vi "Set Rx Monitor Properties.vi"(8 "error in":errorcluster, 10 "session_rx_monitor":T2 {"Strobe" items=["FDX_MON_STROBE_DIS", "FDX_MON_STROBE_STOP", "FDX_MON_STROBE_START"]; "CaptureMode" items=["FDX_MON_SINGLE ", "FDX_MON_CONTINUOUS", "FDX_MON_SELECTIVE", "FDX_MON_RECORDING", "FDX_MON_REROS", "FDX_MON_HMU"]; "DefaultCronoMode" items=["FDX_RX_DEFAULT_ENA_CNT", "FDX_RX_DEFAULT_MON_ENA_ALL", "FDX_RX_DEFAULT_MON_ENA_GOOD"]}, 11 "custom device ref in":T1 format="%.0x") -> (0 "error out":errorcluster, 3 "custom device ref out":T1 format="%.0x")   [LabVIEW 2020, in "AIM ARINC 664 Scripting.lvlib"]
uses:
  AIM ARINC 664 Scripting.lvlib
  <vilib>/NI VeriStand/Custom Device API/Custom Device API.lvlib
  <vilib>/NI VeriStand/Custom Device API/Set Item Property (U32).vi
  Constants.vi
  <vilib>/NI VeriStand/Custom Device API/Custom Device Item Ref.ctl
  Shared/session_rx_monitor.ctl
  Import/AIM ARINC 664 Import.lvlib
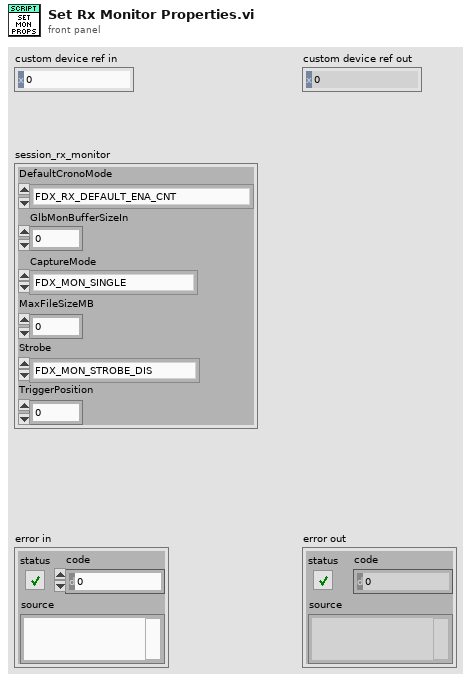
[diagram p1: front panel]
types:
  T1 = typedef "Custom Device API.lvlib/Custom Device Item Ref.ctl" = u64
  T2 = typedef "AIM ARINC 664 Import.lvlib/session_rx_monitor.ctl" = cluster{"DefaultCronoMode":u32, "GlbMonBufferSizeIn":u32, "CaptureMode":u32, "MaxFileSizeMB":u32, "Strobe":u32, "TriggerPosition":u32}
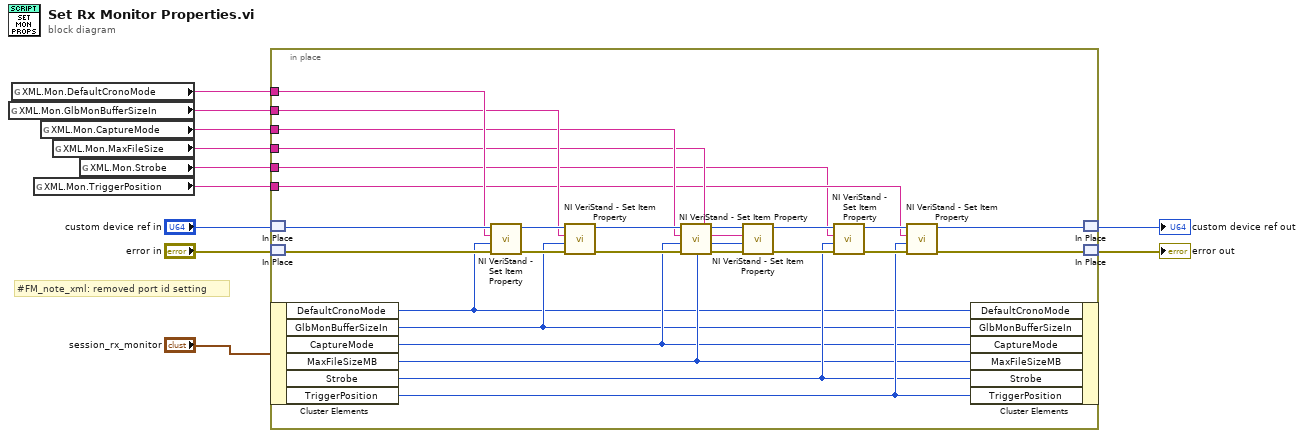
[diagram p0: block diagram]
diagram:
  # "#FM_note_xml: removed port id setting"
  n1 = global read "Constants.vi" "XML.Mon.GlbMonBufferSizeIn"() -> (w5:string)
  n2 = global read "Constants.vi" "XML.Mon.DefaultCronoMode"() -> (w6:string)
  n3 = global read "Constants.vi" "XML.Mon.TriggerPosition"() -> (w2:string)
  n4 = global read "Constants.vi" "XML.Mon.CaptureMode"() -> (w4:string)
  n5 = global read "Constants.vi" "XML.Mon.MaxFileSize"() -> (w3:string)
  n6 = global read "Constants.vi" "XML.Mon.Strobe"() -> (w1:string)
  n7 = in-place {
    in-place-border: w6 -> [w17]
    in-place-border: w5 -> [w16]
    in-place-border: w4 -> [w15]
    in-place-border: w3 -> [w14]
    in-place-border: w2 -> [w13]
    in-place-border: w1 -> [w12]
    n8 = in-place-match #1("custom device ref in") -> (w37:T1)
    n9 = in-place-match #2("error in") -> (w31:errorcluster)
    n10 = in-place-cluster #3("session_rx_monitor") -> ("DefaultCronoMode"=w19:u32, "GlbMonBufferSizeIn"=w20:u32, "CaptureMode"=w21:u32, "MaxFileSizeMB"=w22:u32, "Strobe"=w23:u32, "TriggerPosition"=w24:u32)
    n11 = call-poly <vilib>:"NI VeriStand - Set Item Property.vi"("error in (no error)"=w31, "Value"=w19, "Property Name"=w17, "Item Ref in"=w37) -> ("error out"=w30:errorcluster, "Item Ref out"=w36:T1)  [unwired: 5 in, 1 out]
    n12 = call-poly <vilib>:"NI VeriStand - Set Item Property.vi"("error in (no error)"=w30, "Value"=w20, "Property Name"=w16, "Item Ref in"=w36) -> ("error out"=w29:errorcluster, "Item Ref out"=w35:T1)  [unwired: 5 in, 1 out]
    n13 = call-poly <vilib>:"NI VeriStand - Set Item Property.vi"("error in (no error)"=w29, "Value"=w21, "Property Name"=w15, "Item Ref in"=w35) -> ("error out"=w28:errorcluster, "Item Ref out"=w34:T1)  [unwired: 5 in, 1 out]
    n14 = call-poly <vilib>:"NI VeriStand - Set Item Property.vi"("error in (no error)"=w28, "Value"=w22, "Property Name"=w14, "Item Ref in"=w34) -> ("error out"=w27:errorcluster, "Item Ref out"=w33:T1)  [unwired: 5 in, 1 out]
    n15 = call-poly <vilib>:"NI VeriStand - Set Item Property.vi"("error in (no error)"=w27, "Value"=w23, "Property Name"=w12, "Item Ref in"=w33) -> ("error out"=w26:errorcluster, "Item Ref out"=w32:T1)  [unwired: 5 in, 1 out]
    n16 = call-poly <vilib>:"NI VeriStand - Set Item Property.vi"("error in (no error)"=w26, "Value"=w24, "Property Name"=w13, "Item Ref in"=w32) -> ("error out"=w25:errorcluster, "Item Ref out"=w18:T1)  [unwired: 5 in, 1 out]
    n17 = in-place-cluster #3("DefaultCronoMode"=w19, "GlbMonBufferSizeIn"=w20, "CaptureMode"=w21, "MaxFileSizeMB"=w22, "Strobe"=w23, "TriggerPosition"=w24) -> ()  [unwired: 1 out]
    n18 = in-place-match #1(w18) -> (→"custom device ref out":T1)
    n19 = in-place-match #2(w25) -> (→"error out":errorcluster)
  }
